vi "Get Unsupported Vector Settings Message.vi"(0 "RFmx VNA Session":refnum<k21>, 1 "Sweep":T1, 5 "Port":string, 7 "DUT Pin":string, 9 "DUT Site":i32, 11 "error in":errorcluster) -> (4 "Error Message":string, 15 "error out":errorcluster)   [LabVIEW 2023, in "RFFixtureCharact.Public.lvlib" / "Vector Abstract Path.lvclass"]
uses:
  Vector Abstract Path.lvclass
  Vector Path Group/Type Definitions/Sweep.ctl
  <vilib>/addons/_RFCalAndCharactDatabase/NI_RFCalAndCharact_Database_API.lvlibp/PXIe5633/Controls/Port Settings.ctl
  <vilib>/addons/_RFCalAndCharactDatabase/NI_RFCalAndCharact_Database_API.lvlibp/PXIe5633/PXIe5633.lvlib
  <resource>/objmgr/RFmxInstr.rc
  Vector Path Group/Vector Path Group.lvclass
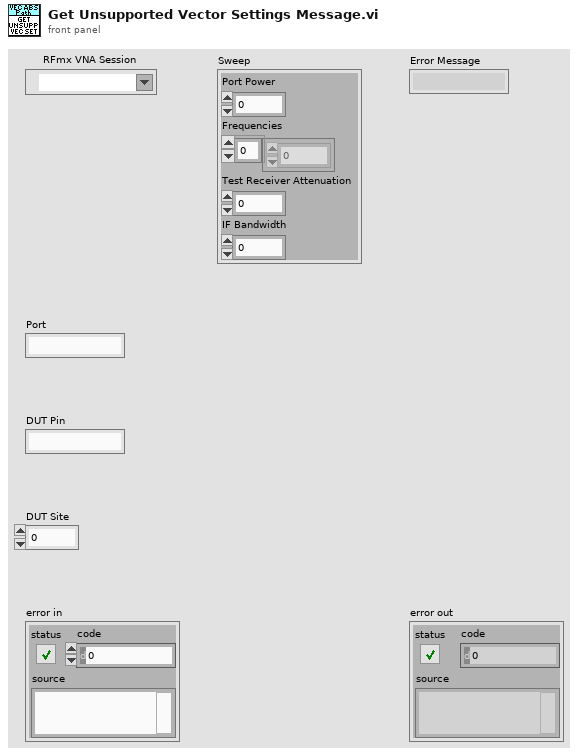
[diagram p1: front panel]
types:
  T1 = typedef "RFFixtureCharact.Public.lvlib/Vector Path Group.lvclass/Sweep.ctl" = cluster{"Port Power":dbl, "Frequencies":dbl[], "Test Receiver Attenuation":dbl, "IF Bandwidth":dbl}
  T2 = typedef "NI_RFCalAndCharact_Database_API.lvlibp/PXIe5633.lvlib/Port Settings.ctl" = cluster{"Port Name":string, "Power Level (dBm)":dbl, "Test Receiver Attenuation (dB)":dbl}
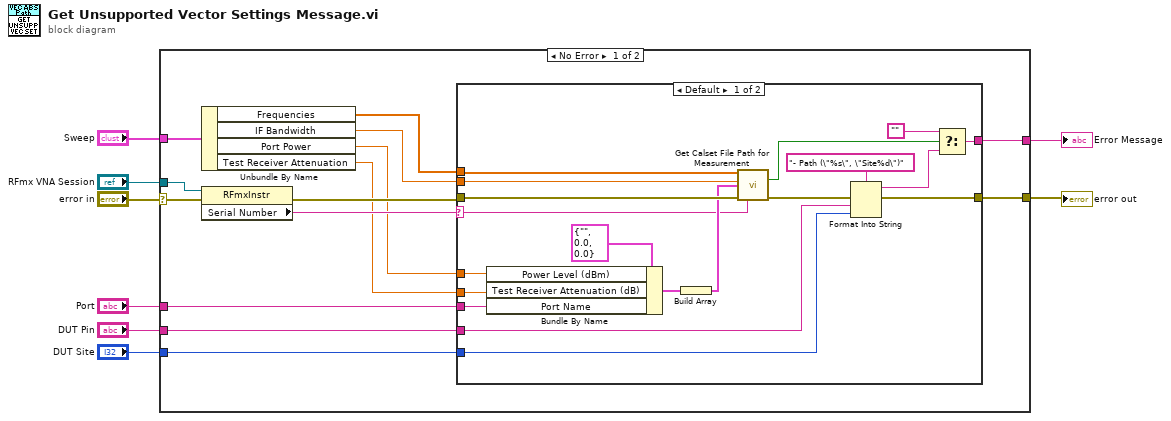
[diagram p0: block diagram]
diagram:
  n1 = case shown="No Error" "error in" {
    selector: "error in" -> [w13 w43]
    tunnel: "DUT Site" -> [w22 _]
    tunnel: [w21 w43] -> w7
    tunnel: [w20 _] -> w6
    tunnel: "DUT Pin" -> [w19 _]
    tunnel: "Port" -> [w10 _]
    tunnel: "Sweep" -> [w14 _]
    tunnel: "RFmx VNA Session" -> [w9 _]
    frame No Error {
      n2 = Unbundle By Name(w14) -> ("Frequencies"=w17:dbl[], "IF Bandwidth"=w18:dbl, "Port Power"=w12:dbl, "Test Receiver Attenuation"=w11:dbl)
      n3 = property class="RFmxInstr"(reference=w9, error in=w13) -> (error out=w15:errorcluster, "Serial Number"=w16:string)  [unwired: 1 out]
      n4 = case shown="Default" w16 {
        selector: w16 -> [w27 _]
        tunnel: w17 -> [w41 _]
        tunnel: w18 -> [w40 _]
        tunnel: w15 -> [w39 w42]
        tunnel: w19 -> [w37 _]
        tunnel: w22 -> [w36 _]
        tunnel: [w25 _] -> w20
        tunnel: [w35 w42] -> w21
        tunnel: w12 -> [w31 _]
        tunnel: w11 -> [w30 _]
        tunnel: w10 -> [w29 _]
        frame Default {
          # "Correction Enabled: True"
          n5 = Bundle By Name(cluster=T2 {"Port Name"="", "Power Level (dBm)"=0.0, "Test Receiver Attenuation (dB)"=0.0} ("Port Settings 2"), "Power Level (dBm)"=w31, "Test Receiver Attenuation (dB)"=w30, "Port Name"=w29) -> (w33:T2)
          n6 = Build Array(w33) -> (w28:T2[])
          n7 = call <vilib>:"Get Calset File Path for Measurement.vi"("Frequency List (Hz)"=w41, "IF Bandwidth (Hz)"=w40, "Port Settings"=w28, "error in"=w39, "VNA Serial Number"=w27) -> ("Found"=w38:bool, "error out"=w23:errorcluster)  [unwired: 8 in, 1 out]
          n8 = Format Into String(format string="- Path (\"%s\", \"Site%d\")", error in=w23, w37, w36) -> (resulting string=w26:string, error out=w35:errorcluster)  [unwired: 1 in]
          n9 = Select(t="", s=w38, f=w26) -> (s? t:f=w25:string)
        }
        frame "" {
          # "Correction Enabled: False"
        }
      }
    }
    frame Error {
    }
  }
  "error out" <- w7
  "Error Message" <- w6
